vi "Window-DestroyWindow.vi"(8 "error in (no error)":errorcluster, 10 "Window Instance":refnum<class "Window.lvclass">, 11 "Engine in":refnum<class "Engine.lvclass">) -> (0 "error out":errorcluster, 3 "Engine out":refnum<class "Engine.lvclass">)   [LabVIEW 2020, in "GLF.lvlib" / "Engine.lvclass"]
uses:
  Engine.lvclass
  Window/Window.lvclass
  Engine.lvclass/Engine.ctl
  Command--enum.ctl
  Command-DestroyWindow--cluster.ctl
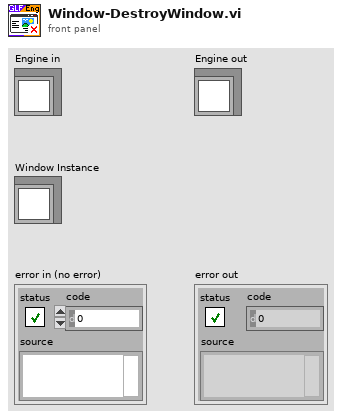
[diagram p1: front panel]
types:
  T1 = typedef "GLF.lvlib/Engine.lvclass/Command-DestroyWindow--cluster.ctl" = cluster{"Window Instance":refnum<class "Window.lvclass">, "Error Return Notifier":refnum<notifier>}
  T2 = typedef "GLF.lvlib/Engine.lvclass/Command--enum.ctl" = enum16{"Quit", "Create Window", "Destroy Window"}
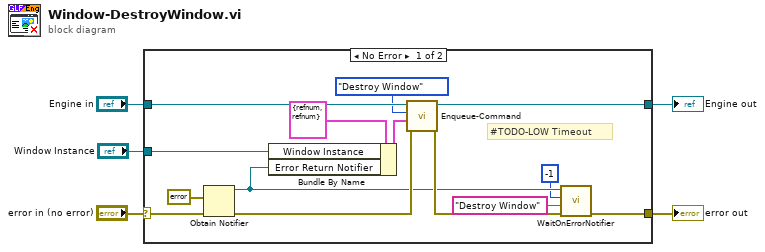
[diagram p0: block diagram]
diagram:
  n1 = case shown="No Error" "error in (no error)" {
    selector: "error in (no error)" -> [w15 w21]
    tunnel: [w6 w21] -> w4
    tunnel: [w18 w20] -> w2
    tunnel: "Engine in" -> [w19 w20]
    tunnel: "Window Instance" -> [w12 _]
    frame No Error {
      # "#TODO-LOW Timeout"
      n2 = Obtain Notifier(notification data type=errorcluster {"status"=FALSE, "code"=0, "source"=""} ("error constant"), error in (no error)=w15) -> (notifier out=w10:refnum<notifier>, error out=w16:errorcluster)  [unwired: 2 in, 1 out]
      n3 = Bundle By Name(cluster=T1 {"Window Instance"=refnum, "Error Return Notifier"=refnum} ("Data"), "Window Instance"=w12, "Error Return Notifier"=w10) -> (w13:T1)
      n4 = call "Enqueue-Command.vi"("error in (no error)"=w16, "Cmd Data"=w13, "Cmd"=Command--enum."Destroy Window", "Engine in"=w19) -> ("error out"=w11:errorcluster, "Engine out"=w18:refnum<class "Engine.lvclass">)  [unwired: 5 in, 1 out]
      n5 = call "WaitOnErrorNotifier.vi"("error in (no error)"=w11, "Timeout additional message (\"\")"="Destroy Window" ("Timeout additional message (\"\")"), "Timeout [ms]"=-1, "Error Notifier"=w10) -> ("error out"=w6:errorcluster)  [unwired: 7 in]
    }
    frame Error {
    }
  }
  "error out" <- w4
  "Engine out" <- w2
